vi "Mcp2210 xfer Spi Data Ex.vi"(5 "SPI Setting":T1={"Chip Setting Selection"=enum."Current Chip Setting(VM)", "Baud Rate"=3000000, "Idle CS Value"=[TRUE, TRUE, TRUE, TRUE, TRUE, TRUE, TRUE, TRUE, TRUE, FALSE, FALSE, FALSE, FALSE, FALSE, FALSE, FALSE, FALSE, FALSE, FALSE, FALSE, FALSE, FALSE, FALSE, FALSE, FALSE, FALSE, FALSE, FALSE, FALSE, FALSE, FALSE, FALSE], "Active CS Value"=[FALSE, FALSE, FALSE, FALSE, FALSE, FALSE, FALSE, FALSE, FALSE, FALSE, FALSE, FALSE, FALSE, FALSE, FALSE, FALSE, FALSE, FALSE, FALSE, FALSE, FALSE, FALSE, FALSE, FALSE, FALSE, FALSE, FALSE, FALSE, FALSE, FALSE, FALSE, FALSE], "CS to Data Delay(us)"=0, "Last Data Byte to CS Delay(us)"=0, "Delay Between Subsequent Data Bytes(us)"=0, "Bytes to Transfer per Transaction"=5, "SPI Mode"=0} {"Baud Rate" format="%.0p"; "SPI Mode" items=["Mode 0", "Mode 1", "Mode 2", "Mode 3"]}, 6 "CS Pin Select":u32(ring) items=["CS0", "CS1", "CS2", "CS3", "CS4", "CS5", "CS6", "CS7", "CS8", "Use Default Setting"], 7 "length":i32, 8 "error in (no error)":errorcluster, 9 "CS select one time":bool, 10 "Tx Data":u8[](array[numeric]) format="%02x", 11 "handle":i32) -> (0 "error out":errorcluster, 2 "RX Data":u8[](array[numeric]) format="%02x", 3 "handle out":i32, 4 "SPI Setting Out":T1 {"SPI Mode" items=["Mode 0", "Mode 1", "Mode 2", "Mode 3"]; "Baud Rate" format="%.0p"})   [LabVIEW 2015, in "mcp2210.lvlib"]
doc: "This function configures the SPI transfer settings (VM parameters only) and initiate the\nSPI data transfer. Basically, this API combines the Mcp2210_SetSPIConfig() and Mcp2210_xferSpiData()\nfunction calls. Also, this function allows the user to specify which GPIO pins to be configured as\nSPI chip select, but it is assumed that the other GPIO pins configuration is already done, either as\npower-up default settings or through the use of Mcp2210_SetGpioConfig() or the other GPIO related API.\nIf the function call succeeds (returns E_SUCCESS), the parameters listed below as \"Inputs/outputs\"\ncontain the configuration values used by device. In some cases, the values are derived from the user\nsupplied ones, being adapted to the device capabilities (e.g. the baudRate).\nPlease note that these changes are not reverted at the end of the SPI data transfer but\nremain in effect until a new GPIO/SPI configuration change is initiated by the user.\nMind that, if there is already an SPI transfer in progress, the configuration change is not accepted\nand the API returns E_ERR_SPI_CFG_ABORT error.\nThis API can also reverse the effect of the GP8 firmware error: when GP8 is set as GPIO \"out\",\nthe SPI transfer command is changing it to GPIO \"in\". The user has the option to skip this fix if the\napplication execution speed gain is relevant.\nParameters:\nInputs:\n- void *handle - The pointer to the device handle. Cannot be NULL.\n- unsigned char *pdataTx - data buffer to be transmitted. Cannot be NULL.\nThe user must ensure that buffer size matches the SPI transfer\nsize setting.\n- unsigned int csmask - bit mask indicating which GPIO pins must be active chip select\n(CS) pins for the SPI transfer.\nbit31 - ... - - bit8 bit0\nGP8CE x ... x x CS8 CS7 CS6 CS5 CS4 CS3 CS2 CS1 CS0\n- A bit value of '1' configures the GPIO pins as CS\n(alternate function 1) during the SPI data transfer.\nA bit value of 0 configures the pins as GPIO (standard function)\nexcept the pins which are configuration as\ndedicated function (alternate function 2).\nThe GPIO direction and default values must be already configured\nas needed either as power-up defaults or with prior use of\nMcp2210_SetGpioConfig().\n- If all CS[0..8] bit values are '0', current GPIO configuration\nis preserved.\n- If csmask[31] bit (GP8CE) is set ('1'), the GP8 errata is\nignored, assuming that user application is not affected by the\nGP8 pin being reconfigured as GPIO \"input\" after the SPI\ntransfer command.\nOutput:\n- unsigned char *pdataRx - receive data buffer. Cannot be NULL.\nThe user must ensure that buffer size matches the SPI transfer\nsize setting.\nInputs / Outputs:\n- unsigned int *pbaudRate - transfer speed. Cannot be NULL.\n- unsigned int *ptxferSize - Bytes to Transfer per SPI Transaction.\n- 16-bit value => max value is (2^16)-1.\n- Cannot be NULL.45\n- unsigned int *pidleCsVal - IDLE chip select value. Cannot be NULL.\nbit31 - - - - bit8 bit0\nx x ... x x CS8 CS7 CS6 CS5 CS4 CS3 CS2 CS1 CS0\n- unsigned int *pactiveCsVal - Active Chip Select Value. Cannot be NULL.\nbit31 - - - - bit8 bit0\nx x ... x x CS8 CS7 CS6 CS5 CS4 CS3 CS2 CS1 CS0\n- unsigned int *pCsToDataDly - Chip Select to Data Delay (quanta of 100 us)\n- 16-bit value => max value is (2^16-1).\n- Cannot be NULL.\n- unsigned int *pdataToCsDly - Last Data Byte to CS (de-asserted) Delay (quanta of 100 us)\n- 16-bit value => max value is (2^16)-1.\n- Cannot be NULL.\n- unsigned int *pdataToDataDly - Delay Between Subsequent Data Bytes (quanta of 100 us)\n- 16-bit value => max value is (2^16)-1.\n- Cannot be NULL.\n- unsigned char *pspiMd - SPI Mode. Cannot be NULL.\nValid values are:\n- MCP2210_SPI_MODE0\n- MCP2210_SPI_MODE1\n- MCP2210_SPI_MODE2\n- MCP2210_SPI_MODE3\nReturns:\n- 0 for success: E_SUCCESS\n- negative error code: E_ERR_NULL, E_ERR_INVALID_HANDLE_VALUE, E_ERR_INVALID_PARAMETER\nE_ERR_HID_TIMEOUT, E_ERR_HID_RW_FILEIO, E_ERR_UNKOWN_ERROR\nE_ERR_CMD_ECHO, E_ERR_CMD_FAILED\nE_ERR_SPI_CFG_ABORT, E_ERR_SPI_TIMEOUT, E_ERR_SPI_EXTERN_MASTER,\nE_ERR_SPI_RX_INCOMPLETE\n\nMCP2210_DLL_UM_API int __stdcall Mcp2210_xferSpiDataEx(void *handle, unsigned char *pdataTx, unsigned char *pdataRx,\n unsigned int *pbaudRate, unsigned int *ptxferSize, unsigned int csmask,\n unsigned int *pidleCsVal, unsigned int *pactiveCsVal, unsigned int *pCsToDataDly,\n unsigned int *pdataToCsDly, unsigned int *pdataToDataDly, unsigned char *pspiMd);"
uses:
  <userlib>/mcp2210/mcp2210.lvlib
  <userlib>/mcp2210/mcp2210_dll_um_x86.dll
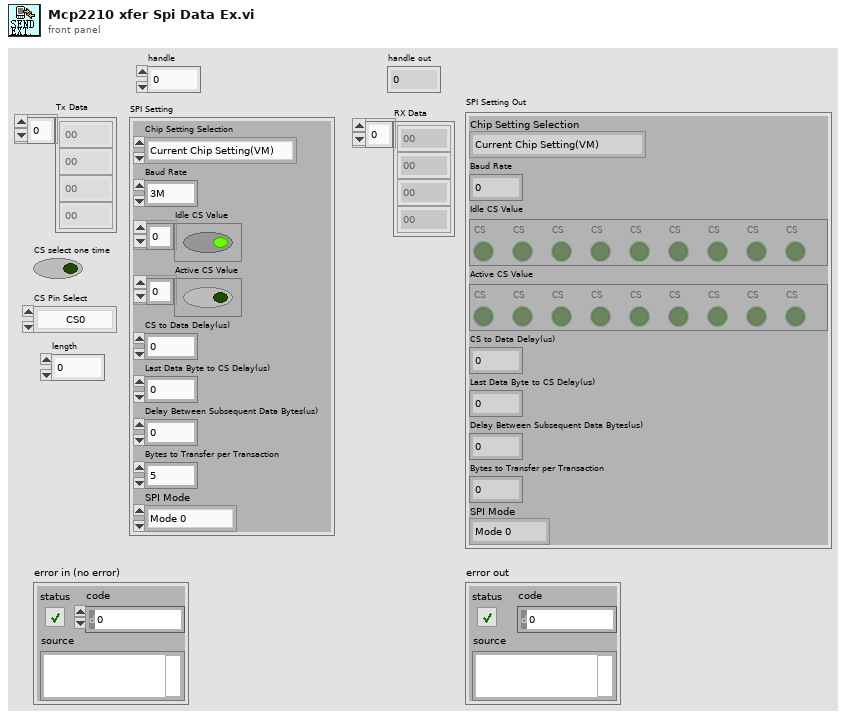
[diagram p1: front panel]
types:
  T1 = cluster{"Chip Setting Selection":enum8{"Current Chip Setting(VM)", "Power-up Chip Setting(NVRAM)"}, "Baud Rate":u32, "Idle CS Value":bool[], "Active CS Value":bool[], "CS to Data Delay(us)":u32, "Last Data Byte to CS Delay(us)":u32, "Delay Between Subsequent Data Bytes(us)":u32, "Bytes to Transfer per Transaction":u32, "SPI Mode":u8}
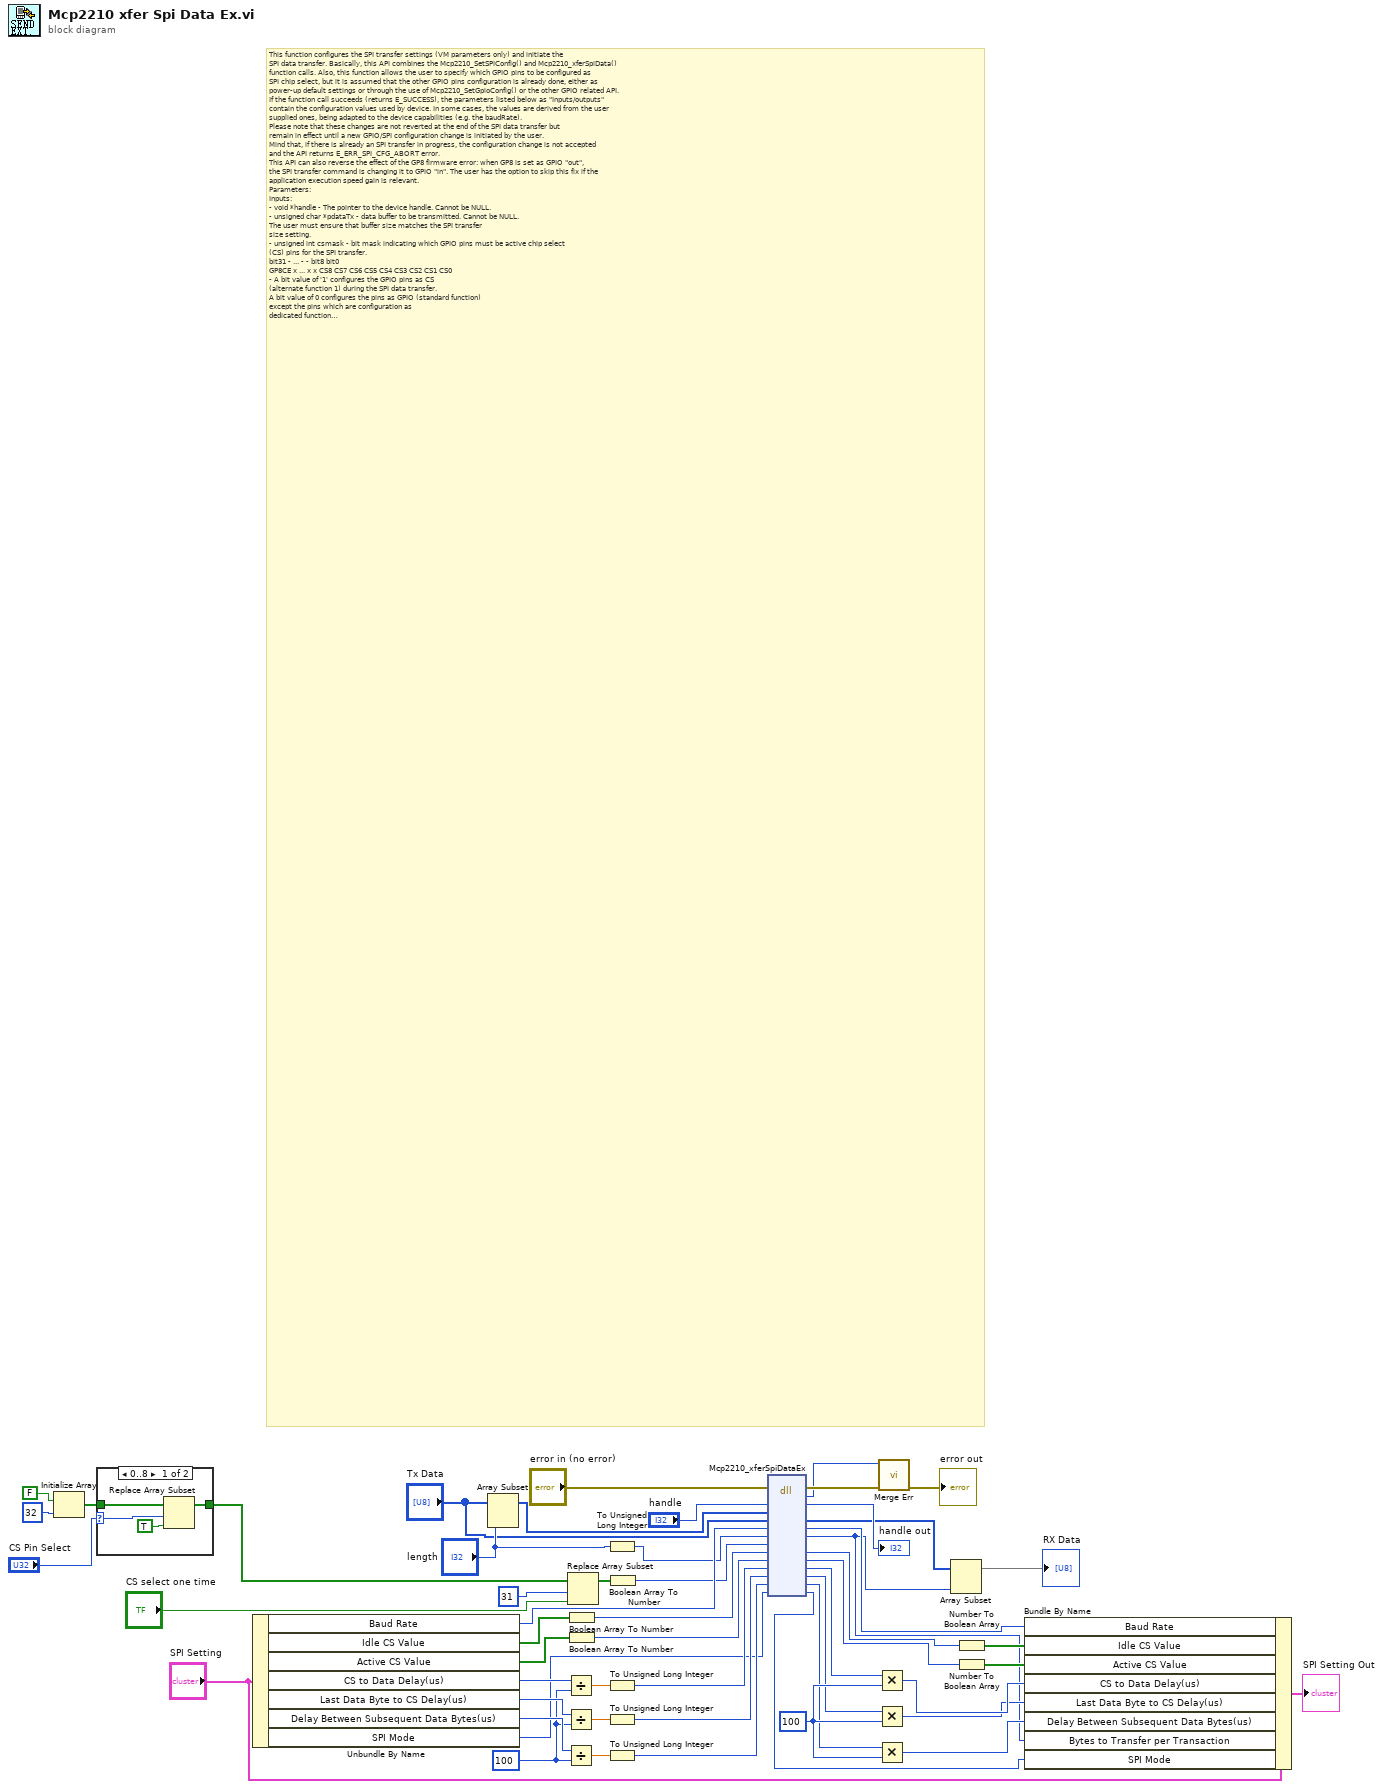
[diagram p0: block diagram]
diagram:
  w13 = u32 100 ("y")
  w26 = u32 100 ("y")
  # "This function configures the SPI transfer settings (VM parameters only) and initiate the\nSPI data transfer. Basically, this API combines the Mcp2210_SetSPIConfig() and Mcp2210_xferSpiData()\nfunction calls. Also, this function allows the user to specify which GPIO pins to be configured as\nSPI chip select, but it is assumed that the other GPIO pins configuration is already done, either as\npower-up default settings or through the use of Mcp2210_SetGpioConfig() or the other GPIO related API.\nIf the function call succeeds (returns E_SUCCESS), the parameters listed below as \"Inputs/outputs\"\ncontain the configuration values used by device. In some cases, the values are derived from the user\nsupplied ones, being adapted to the device capabilities (e.g. the baudRate).\nPlease note that these changes are not reverted at the end of the SPI data transfer but\nremain in effect until a new GPIO/SPI configuration change is initiated by the user.\nMind that, if there is already an SPI transfer in progress, the configuration change is not accepted\nand the API returns E_ERR_SPI_CFG_ABORT error.\nThis API can also reverse the effect of the GP8 firmware error: when GP8 is set as GPIO \"out\",\nthe SPI transfer command is changing it to GPIO \"in\". The user has the option to skip this fix if the\napplication execution speed gain is relevant.\nParameters:\nInputs:\n- void *handle - The pointer to the device handle. Cannot be NULL.\n- unsigned char *pdataTx - data buffer to be transmitted. Cannot be NULL.\nThe user must ensure that buffer size matches the SPI transfer\nsize setting.\n- unsigned int csmask - bit mask indicating which GPIO pins must be active chip select\n(CS) pins for the SPI transfer.\nbit31 - ... - - bit8 bit0\nGP8CE x ... x x CS8 CS7 CS6 CS5 CS4 CS3 CS2 CS1 CS0\n- A bit value of '1' configures the GPIO pins as CS\n(alternate function 1) during the SPI data transfer.\nA bit value of 0 configures the pins as GPIO (standard function)\nexcept the pins which are configuration as\ndedicated function (alternate function 2).\nThe GPIO direction and default values must be already configured\nas needed either as power-up defaults or with prior use of\nMcp2210_SetGpioConfig().\n- If all CS[0..8] bit values are '0', current GPIO configuration\nis preserved.\n- If csmask[31] bit (GP8CE) is set ('1'), the GP8 errata is\nignored, assuming that user application is not affected by the\nGP8 pin being reconfigured as GPIO \"input\" after the SPI\ntransfer command.\nOutput:\n- unsigned char *pdataRx - receive data buffer. Cannot be NULL.\nThe user must ensure that buffer size matches the SPI transfer\nsize setting.\nInputs / Outputs:\n- unsigned int *pbaudRate - transfer speed. Cannot be NULL.\n- unsigned int *ptxferSize - Bytes to Transfer per SPI Transaction.\n- 16-bit value => max value is (2^16)-1.\n- Cannot be NULL.45\n- unsigned int *pidleCsVal - IDLE chip select value. Cannot be NULL.\nbit31 - - - - bit8 bit0\nx x ... x x CS8 CS7 CS6 CS5 CS4 CS3 CS2 CS1 CS0\n- unsigned int *pactiveCsVal - Active Chip Select Value. Cannot be NULL.\nbit31 - - - - bit8 bit0\nx x ... x x CS8 CS7 CS6 CS5 CS4 CS3 CS2 CS1 CS0\n- unsigned int *pCsToDataDly - Chip Select to Data Delay (quanta of 100 us)\n- 16-bit value => max value is (2^16-1).\n- Cannot be NULL.\n- unsigned int *pdataToCsDly - Last Data Byte to CS (de-asserted) Delay (quanta of 100 us)\n- 16-bit value => max value is (2^16)-1.\n- Cannot be NULL.\n- unsigned int *pdataToDataDly - Delay Between Subsequent Data Bytes (quanta of 100 us)\n- 16-bit value => max value is (2^16)-1.\n- Cannot be NULL.\n- unsigned char *pspiMd - SPI Mode. Cannot be NULL.\nValid values are:\n- MCP2210_SPI_MODE0\n- MCP2210_SPI_MODE1\n- MCP2210_SPI_MODE2\n- MCP2210_SPI_MODE3\nReturns:\n- 0 for success: E_SUCCESS\n- negative error code: E_ERR_NULL, E_ERR_INVALID_HANDLE_VALUE, E_ERR_INVALID_PARAMETER\nE_ERR_HID_TIMEOUT, E_ERR_HID_RW_FILEIO, E_ERR_UNKOWN_ERROR\nE_ERR_CMD_ECHO, E_ERR_CMD_FAILED\nE_ERR_SPI_CFG_ABORT, E_ERR_SPI_TIMEOUT, E_ERR_SPI_EXTERN_MASTER,\nE_ERR_SPI_RX_INCOMPLETE\n\nMCP2210_DLL_UM_API int __stdcall Mcp2210_xferSpiDataEx(void *handle, unsigned char *pdataTx, unsigned char *pdataRx,\n                                                       unsigned int *pbaudRate, unsigned int *ptxferSize, unsigned int csmask,\n                                                       unsigned int *pidleCsVal, unsigned int *pactiveCsVal, unsigned int *pCsToDataDly,\n                                                       unsigned int *pdataToCsDly, unsigned int *pdataToDataDly, unsigned char *pspiMd);"
  n1 = Initialize Array(FALSE, 32 ("dimension size")) -> (w47:bool[])
  n2 = case shown="0..8" "CS Pin Select" {
    selector: "CS Pin Select" -> [w56 _]
    tunnel: w47 -> [w57 w58]
    tunnel: [w54 w58] -> w48
    frame 0..8 {
      n3 = Replace Array Subset(array=w57, new element=TRUE ("new element/subarray"), index=w56) -> (w54:bool[])
    }
    frame 9, Default {
    }
  }
  n4 = Unbundle By Name("SPI Setting") -> ("Baud Rate"=w49:u32, "Idle CS Value"=w39:bool[], "Active CS Value"=w38:bool[], "CS to Data Delay(us)"=w34:u32, "Last Data Byte to CS Delay(us)"=w31:u32, "Delay Between Subsequent Data Bytes(us)"=w27:u32, "SPI Mode"=w4:u8)
  n5 = Array Subset(array="Tx Data", length="length") -> (w7:u8[])  [unwired: 1 in]
  n6 = Divide(x=w34, y=w26) -> (x/y=w33:dbl)
  n7 = Divide(x=w31, y=w26) -> (x/y=w30:dbl)
  n8 = Divide(x=w27, y=w26) -> (x/y=w28:dbl)
  n9 = Boolean Array To Number(Boolean array=w39) -> (number=w37:u32)
  n10 = Boolean Array To Number(Boolean array=w38) -> (number=w35:u32)
  n11 = Replace Array Subset(array=w48, new element="CS select one time", index=31) -> (w41:bool[])
  n12 = To Unsigned Long Integer(number="length") -> (unsigned 32bit integer=w36:u32)
  n13 = To Unsigned Long Integer(number=w33) -> (unsigned 32bit integer=w32:u32)
  n14 = To Unsigned Long Integer(number=w30) -> (unsigned 32bit integer=w29:u32)
  n15 = To Unsigned Long Integer(number=w28) -> (unsigned 32bit integer=w25:u32)
  n16 = Boolean Array To Number(Boolean array=w41) -> (number=w40:u32)
  n17 = dll-call lib="D:/LabVIEW 2015/user.lib/mcp2210/mcp2210_dll_um_x86.*" fn="Mcp2210_xferSpiDataEx"(error in="error in (no error)", "handle"="handle", "pdataTx"=w7, "pdataRx"="Tx Data", "pbaudRate"=w49, "ptxferSize"=w36, "csmask"=w40, "pidleCsVal"=w37, "pactiveCsVal"=w35, "pCsToDataDly"=w32, "pdataToCsDly"=w29, "pdataToDataDly"=w25, "pspiMd"=w4) -> (error out=w51:errorcluster, "return type"=w50:i32, "handle"=→"handle out":i32, "pdataRx"=w5:u8[], "pbaudRate"=w17:u32, "ptxferSize"=w1:u32, "pidleCsVal"=w16:u32, "pactiveCsVal"=w15:u32, "pCsToDataDly"=w14:u32, "pdataToCsDly"=w12:u32, "pdataToDataDly"=w11:u32, "pspiMd"=w3:u8)  [unwired: 4 in, 1 out]
  n18 = Multiply(x=w14, y=w13) -> (x*y=w20:u32)
  n19 = Multiply(x=w12, y=w13) -> (x*y=w19:u32)
  n20 = Multiply(x=w11, y=w13) -> (x*y=w18:u32)
  n21 = call <userlib>:"Merge Err.vi"("error in (no error)"=w51, "return type"=w50) -> ("error out"=→"error out":errorcluster)  [unwired: 9 in]
  n22 = Array Subset(array=w5, length=w1) -> (→"RX Data":u8[])  [unwired: 1 in]
  n23 = Number To Boolean Array(number=w16) -> (Boolean array=w22:bool[])
  n24 = Number To Boolean Array(number=w15) -> (Boolean array=w21:bool[])
  n25 = Bundle By Name(cluster="SPI Setting", "Baud Rate"=w17, "Idle CS Value"=w22, "Active CS Value"=w21, "CS to Data Delay(us)"=w20, "Last Data Byte to CS Delay(us)"=w19, "Delay Between Subsequent Data Bytes(us)"=w18, "Bytes to Transfer per Transaction"=w1, "SPI Mode"=w3) -> (→"SPI Setting Out":T1)
